vi "SetCC.vi"(8 "error in (no error)":errorcluster, 9 "Chan":i32, 10 "CC":dbl, 11 "reference in":refnum<class "PSU_Keysight_34951A.lvclass">) -> (0 "error out":errorcluster, 3 "reference in":refnum<class "PSU_Keysight_34951A.lvclass">)   [LabVIEW 2022 SP3, in "PSU_Keysight_34951A.lvlib" / "PSU_Keysight_34951A.lvclass"]
uses:
  PSU_Keysight_34951A.lvclass
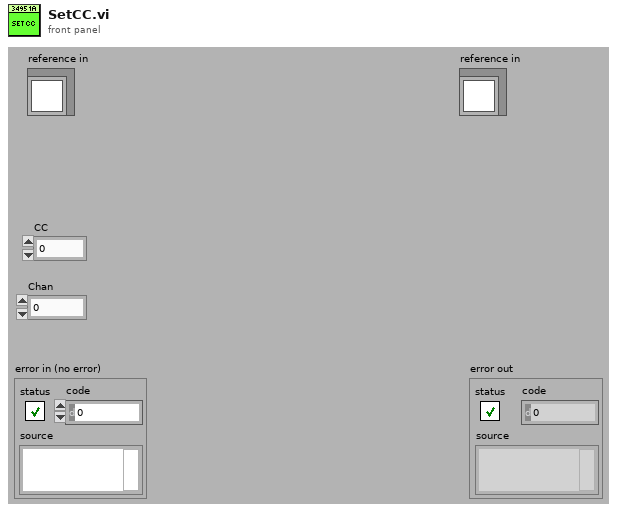
[diagram p1: front panel]
types:
  T1 = typedef "PSU_Keysight_34951A.lvlib/PSU_Keysight_34951A.lvclass/ObjectAttributes.ctl" = cluster{"Config":T2, "VISA res":refnum<visa-resource-name>, "Enabled":bool[], "V":dbl[], "I":dbl[], "Source Type":enum16{"Voltage", "Current"}[]}
  T2 = typedef "PSU_Keysight_34951A.lvlib/PSU_Keysight_34951A.lvclass/Config.ctl" = cluster{"VISA":refnum<visa-resource-name>, "Slot":i32}
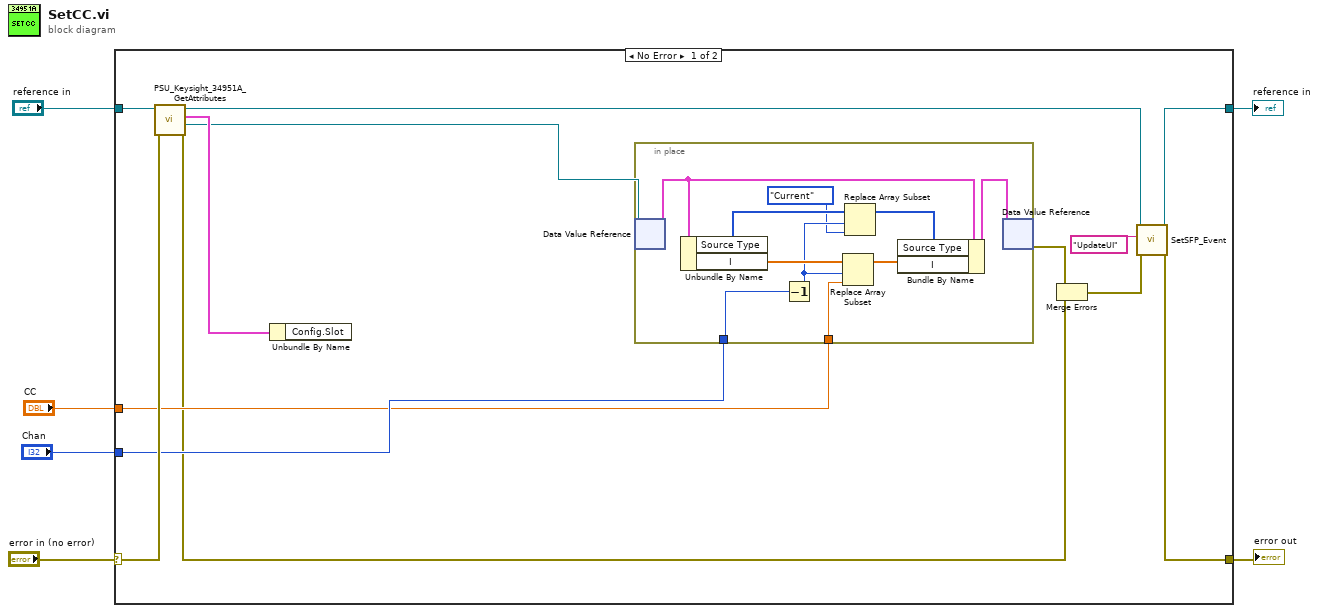
[diagram p0: block diagram]
diagram:
  n1 = case shown="No Error" "error in (no error)" {
    selector: "error in (no error)" -> [w19 w31]
    tunnel: [w12 w31] -> w5
    tunnel: [w13 w30] -> w3
    tunnel: "reference in" -> [w18 w30]
    tunnel: "Chan" -> [w11 _]
    tunnel: "CC" -> [w10 _]
    frame No Error {
      n2 = call "PSU_Keysight_34951A_GetAttributes.vi"("error in (no error)"=w19, "reference in"=w18) -> ("error out"=w7:errorcluster, "DataRef"=w9:refnum<data-value>, "Data"=w17:T1, "reference out"=w14:refnum<class "PSU_Keysight_34951A.lvclass">)  [unwired: 6 in]
      n3 = Unbundle By Name(w17) -> ()  [unwired: 1 out]
      n4 = in-place {
        in-place-border: w11 -> [w27]
        in-place-border: w10 -> [w24]
        n5 = in-place-dvr #1(w9) -> (w28:T1)  [unwired: 1 out]
        n6 = Unbundle By Name(w28) -> ("Source Type"=w23:enum16{"Voltage", "Current"}[], "I"=w26:dbl[])
        n7 = Decrement(x=w27) -> (x-1=w21:i32)
        n8 = Replace Array Subset(array=w26, new element=w24, index=w21) -> (w25:dbl[])
        n9 = Replace Array Subset(array=w23, new element=enum16{"Voltage", "Current"}."Current" ("new element/subarray"), index=w21) -> (w22:enum16{"Voltage", "Current"}[])
        n10 = Bundle By Name(cluster=w28, "Source Type"=w22, "I"=w25) -> (w29:T1)
        n11 = in-place-dvr #1(w29) -> (w16:errorcluster)  [unwired: 1 out]
      }
      n12 = Merge Errors(w16, w7) -> (w15:errorcluster)
      n13 = call-dynamic "SetSFP_Event.vi"("error in (no error)"=w15, "msg"="UpdateUI" ("Ancestor"), "reference in"=w14) -> ("error out"=w12:errorcluster, "reference out"=w13:refnum<class "PSU_Keysight_34951A.lvclass">)  [unwired: 7 in]
    }
    frame Error {
    }
  }
  "error out" <- w5
  "reference in" <- w3
